vi "simulado ctl.vi"(8 "error in (no error)":errorcluster, 9 "Visa com port":refnum<visa-resource-name>, 10 "Serial Device Brand":T1, 11 "Simulado in":refnum<class "Simulado.lvclass">) -> (0 "error out":errorcluster, 3 "Simulado out":refnum<class "Simulado.lvclass">)   [LabVIEW 2020, in "Simulado.lvclass"]
uses:
  Simulado.lvclass
  Combo box/serial device brand.ctl
  Abstracts/Serial Device/Serial Device.lvclass
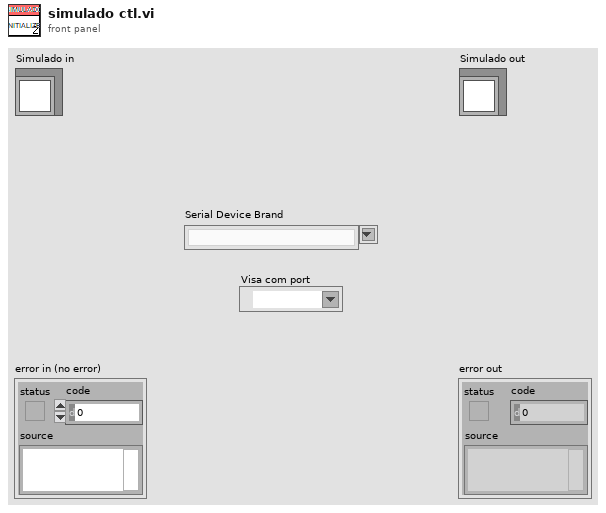
[diagram p1: front panel]
types:
  T1 = typedef "Serial Device.lvclass/serial device brand.ctl" = string
  T2 = enum16{"reset parameters", "Get parameters", "Set parameter"}
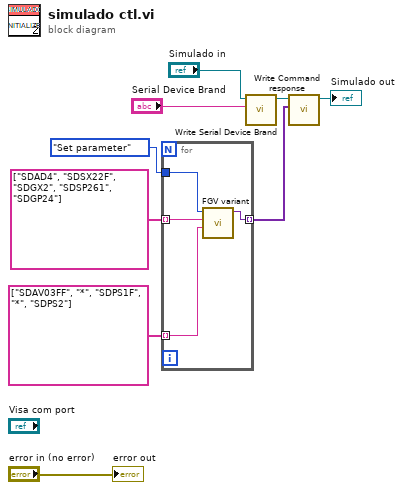
[diagram p0: block diagram]
diagram:
  n1 = for {
    tunnel: T2."Set parameter" ("Functions") -> [w13]
    tunnel: string[] ["SDAD4", "SDSX22F", "SDGX2", "SDSP261", "SDGP24"] ("Command") -> [w12] mode=indexing
    tunnel: string[] ["SDAV03FF", "*", "SDPS1F", "*", "SDPS2"] ("Response to save") -> [w11] mode=indexing
    tunnel: [w10] -> w1 mode=indexing
    n2 = call "FGV variant.vi"("Response to save"=w11, "Command"=w12, "Functions"=w13) -> ("Variant"=w10:variant)  [unwired: 7 in, 1 out]
  }
  n3 = call-dynamic "Write Serial Device Brand.vi"("Serial Device Brand"="Serial Device Brand", "Serial Device in"="Simulado in") -> ("Serial Device out"=w3:refnum<class "Simulado.lvclass">)  [unwired: 8 in, 1 out]
  n4 = call-dynamic "Write Command response.vi"("Command response"=w1, "Simulado in"=w3) -> ("Simulado out"=→"Simulado out":refnum<class "Simulado.lvclass">)  [unwired: 8 in, 1 out]
  "error out" <- "error in (no error)"
